vi "Actuators Get Jog Step.vi"(0 "Notifier Name":string, 11 "Error In":errorcluster) -> (4 "Notifier Name Out":string, 8 "Jog Step":dbl[](array[numeric]), 15 "Error Out":errorcluster)   [LabVIEW 2020]
uses:
  Actuators Controls/Actuators Note Type.ctl
  Actuators Controls/Actuators Actions.ctl
  49aba3af-00be-4f7a-b524-f0c494369c45.vi
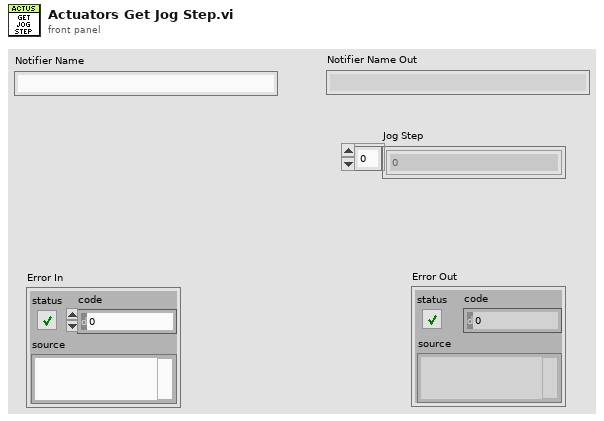
[diagram p1: front panel]
types:
  T1 = typedef "Actuators Note Type.ctl" = cluster{"Actions":T2, "Cmd Received ":bool, "Setpoint":dbl[], "Position":dbl[], "Channel":i32[], "Jog Step":dbl[], "Velocity":dbl[], "Acceleration":dbl[], "Status Bits":u32[]}
  T2 = typedef "Actuators Actions.ctl" = enum16{"Nothing", "Get Position", "Get Acceleration", "Get Velocity", "Get Jog Step", "Set Acceleration", "Set Velocity", "Set Jog Step", "Move Absolute", "Move Relative", "Jog Forward", "Jog Reverse", "Halt", "Quit"}
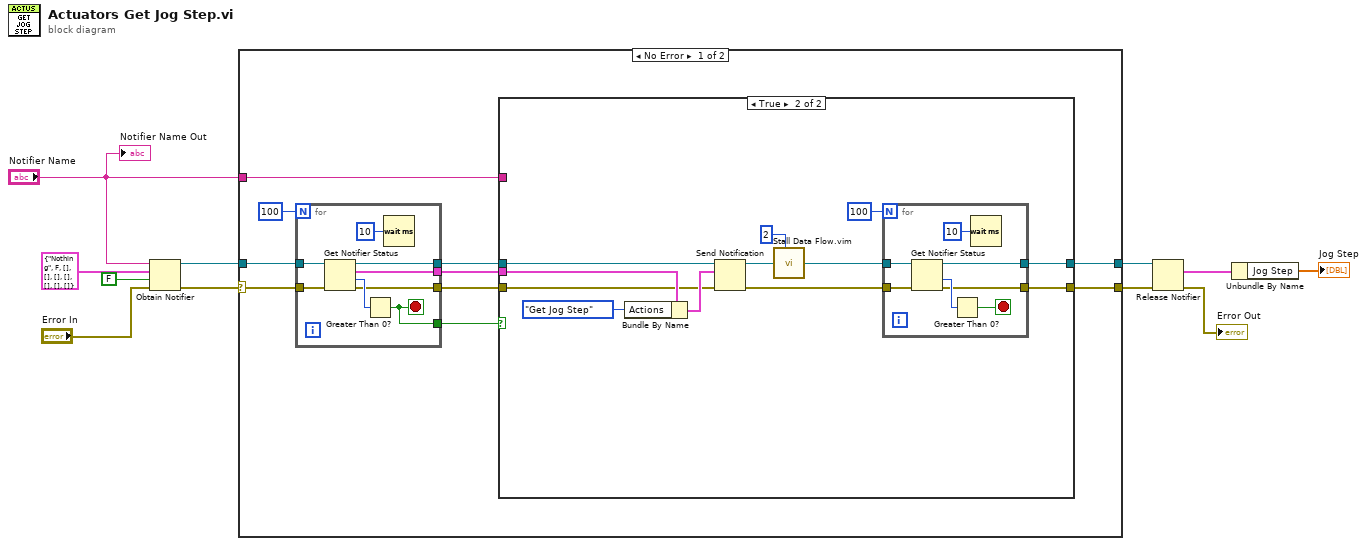
[diagram p0: block diagram]
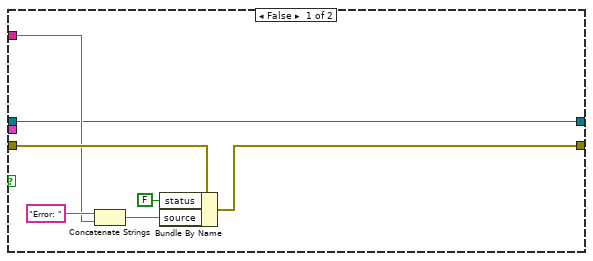
[diagram p2: hidden frame]
diagram:
  n1 = Obtain Notifier(name (unnamed)="Notifier Name", notification data type=T1 {"Actions"=enum."Nothing", "Cmd Received "=FALSE, "Setpoint"=[], "Position"=[], "Channel"=[], "Jog Step"=[], "Velocity"=[], "Acceleration"=[], "Status Bits"=[]} ("Actuators Note"), create if not found? (T)=FALSE, error in (no error)="Error In") -> (notifier out=w7:refnum<notifier>, error out=w10:errorcluster)  [unwired: 1 out]
  n2 = case shown="No Error" w10 {
    selector: w10 -> [w19 w56]
    tunnel: w7 -> [w20 w57]
    tunnel: "Notifier Name" -> [w14 _]
    tunnel: [w13 w57] -> w6
    tunnel: [w12 w56] -> w5
    frame No Error {
      n3 = for {
        N: 100 -> [_]
        tunnel: [w54] -> w16
        tunnel: w20 -> [w55]
        tunnel: [w53] -> w17
        tunnel: w19 -> [w50]
        tunnel: [w49] -> w18
        tunnel: [w48] -> w15
        stop <- w49 stop-if-true
        n4 = Get Notifier Status(notifier=w55, error in (no error)=w50) -> (notifier out=w53:refnum<notifier>, current notification=w54:T1, # waiting=w52:i32, error out=w48:errorcluster)  [unwired: 1 out]
        n5 = Greater Than 0?(x=w52) -> (x > 0?=w49:bool)
        n6 = Wait (ms)(milliseconds to wait=u32 10) -> ()  [unwired: 1 out]
      }
      n7 = case shown="True" w18 {
        tunnel: w17 -> [w23 w40]
        tunnel: w16 -> [_ w39]
        tunnel: w15 -> [w28 w36]
        tunnel: w14 -> [w24 _]
        tunnel: [w23 w31] -> w13
        tunnel: [w22 w32] -> w12
        frame False {
          n8 = Concatenate Strings("Error: " ("source"), w24) -> (w25:string)
          n9 = Bundle By Name(cluster=w28, "status"=FALSE, "source"=w25) -> (w22:errorcluster)
        }
        frame True {
          n10 = Bundle By Name(cluster=w39, "Actions"=Actuators_Actions."Get Jog Step") -> (w37:T1)
          n11 = Send Notification(notification=w37, notifier=w40, error in (no error)=w36) -> (notifier out=w34:refnum<notifier>, error out=w33:errorcluster)
          n12 = call "Stall Data Flow.vim"("value in"=w34, "milliseconds to wait"=u32 2) -> ("value out"=w30:refnum<notifier>)  [unwired: 1 out]
          n13 = for {
            N: 100 -> [_]
            tunnel: w30 -> [w47]
            tunnel: [w46] -> w31
            tunnel: w33 -> [w43]
            tunnel: [w41] -> w32
            stop <- w42 stop-if-true
            n14 = Get Notifier Status(notifier=w47, error in (no error)=w43) -> (notifier out=w46:refnum<notifier>, # waiting=w45:i32, error out=w41:errorcluster)  [unwired: 2 out]
            n15 = Greater Than 0?(x=w45) -> (x > 0?=w42:bool)
            n16 = Wait (ms)(milliseconds to wait=u32 10) -> ()  [unwired: 1 out]
          }
        }
      }
    }
    frame Error {
    }
  }
  n17 = Release Notifier(notifier=w6, error in (no error)=w5) -> (last notification=w2:T1, error out=→"Error Out":errorcluster)  [unwired: 1 in, 1 out]
  n18 = Unbundle By Name(w2) -> ("Jog Step"=→"Jog Step":dbl[])
  "Notifier Name Out" <- "Notifier Name"
